vi "viewlookup.vi"() -> ()   [LabVIEW 2022 SP3]
uses:
  <vilib>/Utility/file.llb/Read From Spreadsheet File (DBL).vi
  <vilib>/Platform/NI_3dgraph.lvlib
  <vilib>/Analysis/NI_AALBase.lvlib
panel:
  in  "Look Up Dimension":i32=40
  in  "Choose Lookup Table":path
  in  "10-31 2":refnum<k7>(container)
  in  "10-13":sgl[][][](array[numeric])=array40x40x40[64000 elements] format="%.6f"
  in  "Index (page)":i32
  in  "PSA Plane":refnum<k7>(container)
  in  "10-31":sgl[][][](array[numeric])=array40x40x40[64000 elements] format="%.6f"
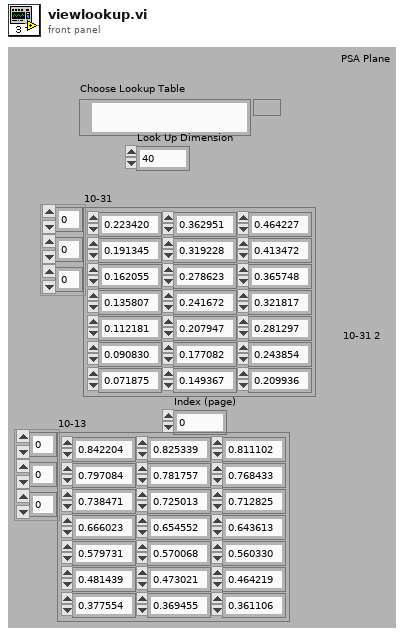
[diagram p1: front panel]
types:
  T1 = cluster{"[0]":dbl, "[1]":dbl, "[2]":dbl, "[3]":dbl, "[4]":dbl, "[5]":dbl, "[6]":dbl, "[7]":dbl}
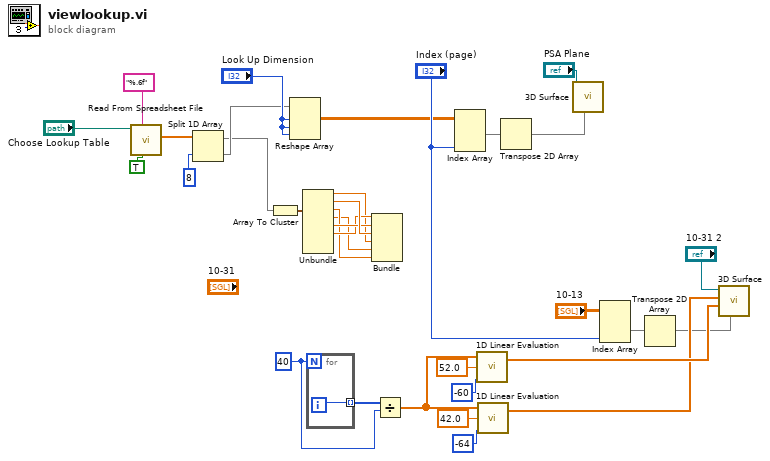
[diagram p0: block diagram]
diagram:
  w25 = 40
  n1 = call-poly <vilib>:"Read From Spreadsheet File.vi"("transpose (no:F)"=TRUE, "format (%.3f)"="%.6f", "file path (dialog if empty)"="Choose Lookup Table") -> ("first row"=w4:dbl[])  [unwired: 1 in, 7 out]
  n2 = Split 1D Array(array=w4, index=8) -> (first subarray=w1:dbl[], second subarray=w2:dbl[])
  n3 = Array To Cluster(array=w1) -> (cluster=w11:T1)
  n4 = Reshape Array(w2, "Look Up Dimension", "Look Up Dimension", "Look Up Dimension") -> (w12:dbl[][][])
  n5 = Unbundle(w11) -> ("[0]"=w5:dbl, "[1]"=w10:dbl, "[2]"=w7:dbl, "[3]"=w6:dbl, "[4]"=w9:dbl, "[5]"=w8:dbl)  [unwired: 2 out]
  n6 = for {
    N: w25 -> [_]
    tunnel: [w34] -> w27 mode=indexing
    i -> [w34]
  }
  n7 = Bundle("[5]"=w8, "[4]"=w9, "[1]"=w10, "[0]"=w5, "[3]"=w6, "[2]"=w7) -> ()  [unwired: 2 out]
  n8 = Divide(x=w27, y=w25) -> (x/y=w26:dbl[])
  n9 = Index Array(array=w12, index (dim 2)="Index (page)") -> (element=w32:dbl[][])  [unwired: 2 in]
  n10 = call <vilib>:"1D Linear Evaluation.vi"("offset"=-60, "scale"=52.0, "X"=w26) -> ("Y[i]=X[i]*a+b"=w19:dbl[])  [unwired: 1 out]
  n11 = call <vilib>:"1D Linear Evaluation.vi"("offset"=-64, "scale"=42.0, "X"=w26) -> ("Y[i]=X[i]*a+b"=w18:dbl[])  [unwired: 1 out]
  n12 = Transpose 2D Array(2D array=w32) -> (transposed array=w20:dbl[][])
  n13 = call <vilib>:"3D Surface.vi"("z matrix"=w20, "3D graph"="PSA Plane") -> ()  [unwired: 1 in, 9 out]
  n14 = Index Array(array="10-13", index (dim 2)="Index (page)") -> (element=w21:sgl[][])  [unwired: 2 in]
  n15 = Transpose 2D Array(2D array=w21) -> (transposed array=w17:sgl[][])
  n16 = call <vilib>:"3D Surface.vi"("z matrix"=w17, "y vector"=w19, "x vector"=w18, "3D graph"="10-31 2") -> ()  [unwired: 1 in, 7 out]
